vi "TelemetryLogger.vi"(6 "Time Stamp":timestamp, 10 "Data":variant, 11 "Sensor:Reading":string) -> ()   [LabVIEW 2014]
uses:
  Type Defs/telemetryReading.ctl
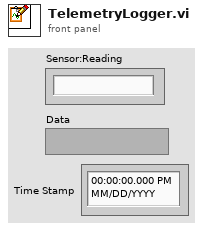
[diagram p1: front panel]
types:
  T1 = typedef "telemetryReading.ctl" = cluster{"Sensor:Reading":string, "Data":variant, "Time Stamp":timestamp}
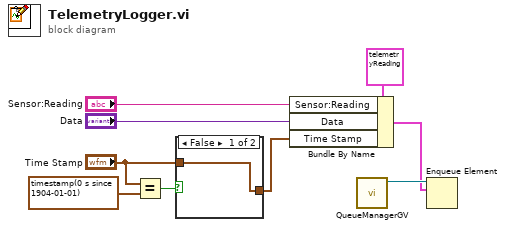
[diagram p0: block diagram]
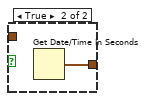
[diagram p2: hidden frame]
diagram:
  n1 = Equal?(x="Time Stamp", y=timestamp(0 s since 1904-01-01) ("Time Stamp")) -> (x = y?=w6:bool)
  n2 = case shown="False" w6 {
    tunnel: [w10 w11] -> w4
    tunnel: "Time Stamp" -> [w10 _]
    frame False {
    }
    frame True {
      n3 = Get Date/Time In Seconds() -> (seconds since 1Jan1904=w11:timestamp)
    }
  }
  n4 = Bundle By Name(cluster=T1 {"Sensor:Reading"="", "Data"=variant, "Time Stamp"=timestamp(3584563538.456057 s since 1904-01-01)} ("Telemetry Reading"), "Sensor:Reading"="Sensor:Reading", "Data"="Data", "Time Stamp"=w4) -> (w1:T1)
  n5 = call "QueueManagerGV.vi"() -> ("Queue"=w2:refnum<queue>)  [unwired: 11 in]
  n6 = Enqueue Element(queue=w2, element=w1) -> ()  [unwired: 2 in, 3 out]
